vi "LAN Config Dynamic DNS.vi"(0 "VISA resource name":refnum<visa-resource-name>, 1 "Hostname":string, 3 "Domain":string, 5 "Node In":string, 9 "Enable (No)":bool, 11 "error in":errorcluster, 12 "Verify (Off)":bool, 13 "Timeout (10000)":u32=10000) -> (4 "VISA resource name out":refnum<visa-resource-name>, 6 "Node Out":string, 14 "Command String":string, 15 "error out":errorcluster)   [LabVIEW 2009, in "Keithley 2600 Series.lvlib"]
uses:
  <instrlib>/Keithley 2600 Series/Keithley 2600 Series.lvlib
  <instrlib>/Keithley 2600 Series/Private/GlobalVariables.vi
panel:
  # "(c) 2008 Keithley Instruments, Inc.  ALL RIGHTS RESERVED."
  # "Enabled Settings"
  # "."
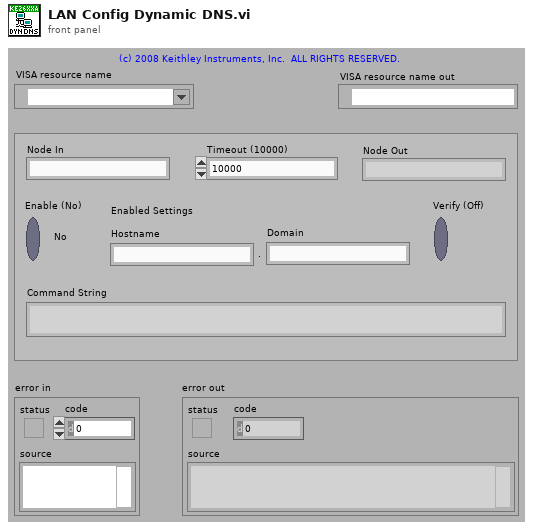
[diagram p1: front panel]
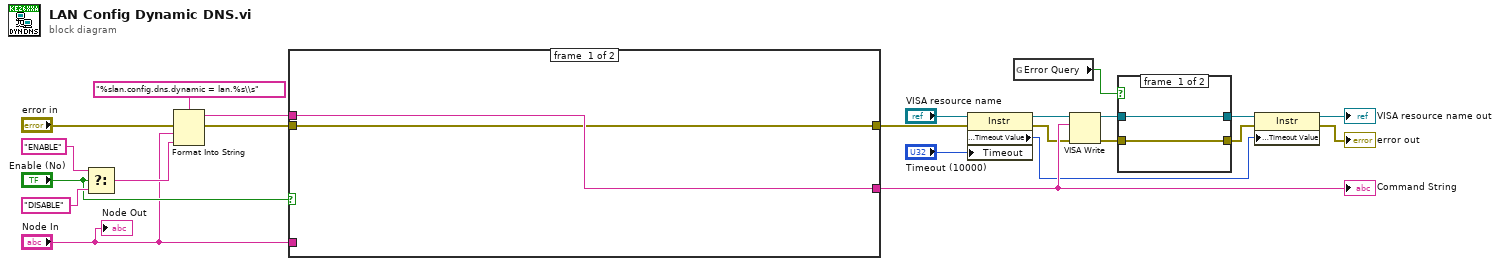
[diagram p0: block diagram]
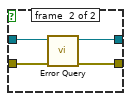
[diagram p2: hidden frame]
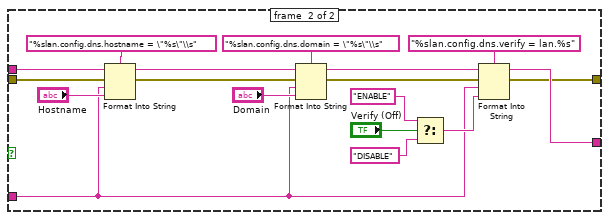
[diagram p3: hidden frame]
diagram:
  n1 = Select(t="ENABLE", s="Enable (No)", f="DISABLE") -> (s? t:f=w20:string)
  n2 = Format Into String(format string="%slan.config.dns.dynamic = lan.%s\\s", error in="error in", "Node In", w20) -> (resulting string=w16:string, error out=w17:errorcluster)  [unwired: 1 in]
  n3 = case shown="True" "Enable (No)" {
    tunnel: w17 -> [w24 w30]
    tunnel: w16 -> [w25 w29]
    tunnel: "Node In" -> [_ w28]
    tunnel: [w25 w27] -> w11
    tunnel: [w24 w26] -> w9
    frame #0 {
    }
    frame #1 {
      n4 = Format Into String(format string="%slan.config.dns.hostname = \"%s\"\\s", initial string=w29, error in=w30, w28, "Hostname") -> (resulting string=w35:string, error out=w37:errorcluster)
      n5 = Format Into String(format string="%slan.config.dns.domain = \"%s\"\\s", initial string=w35, error in=w37, w28, "Domain") -> (resulting string=w34:string, error out=w36:errorcluster)
      n6 = Select(t="ENABLE", s="Verify (Off)", f="DISABLE") -> (s? t:f=w33:string)
      n7 = Format Into String(format string="%slan.config.dns.verify = lan.%s", initial string=w34, error in=w36, w28, w33) -> (resulting string=w27:string, error out=w26:errorcluster)
    }
  }
  "Command String" <- w11
  n8 = property class="Instr"(reference="VISA resource name", error in=w9, "Timeout"="Timeout (10000)") -> (reference out=w8:refnum<visa-resource-name>, error out=w7:errorcluster, "General Settings:Timeout Value"=w1:u32)
  n9 = global read "GlobalVariables.vi" "Error Query"() -> (w14:bool)
  n10 = VISA Write(VISA resource name=w8, write buffer=w11, error in (no error)=w7) -> (VISA resource name out=w13:refnum<visa-resource-name>, error out=w12:errorcluster)  [unwired: 1 out]
  n11 = case shown="True" w14 {
    tunnel: w13 -> [w45 w49]
    tunnel: w12 -> [w44 w48]
    tunnel: [w45 w47] -> w5
    tunnel: [w44 w46] -> w2
    frame #0 {
    }
    frame #1 {
      n12 = call <instrlib>:"Error Query.vi"("error in (no error)"=w48, "VISA resource name"=w49) -> ("error out"=w46:errorcluster, "VISA resource name out"=w47:refnum<visa-resource-name>)  [unwired: 8 out]
    }
  }
  n13 = property class="Instr"(reference=w5, error in=w2, "General Settings:Timeout Value"=w1) -> (reference out=→"VISA resource name out":refnum<visa-resource-name>, error out=→"error out":errorcluster)
  "Node Out" <- "Node In"
